vi "Terminal-Modbus-GetRead.vi"(0 "GuiModbusQRef":refnum<queue>, 11 "error in (no error)":errorcluster caption="错误输入（无错误）") -> (3 "液压子系统":u16[](array[numeric]), 4 "齿轮子系统-PLC":u16[](array[numeric]), 6 "齿轮子系统-数显表":u16[](array[numeric]), 8 "动力子系统-PLC":u16[](array[numeric]), 10 "动力子系统-温度巡检仪":u16[](array[numeric]), 14 "NI工控机":u16[](array[numeric]), 15 "error out":errorcluster caption="错误输出")   [LabVIEW 2014]
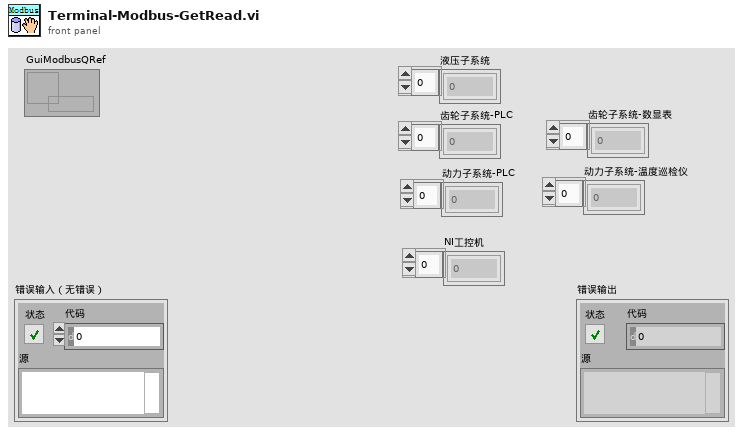
[diagram p1: front panel]
types:
  T1 = cluster{"Transaction ID":u16, "Unit ID":u8, "Starting Address":u16, "Quantity":u16, "Holding Registers":u16[], "Exception Code":u8}
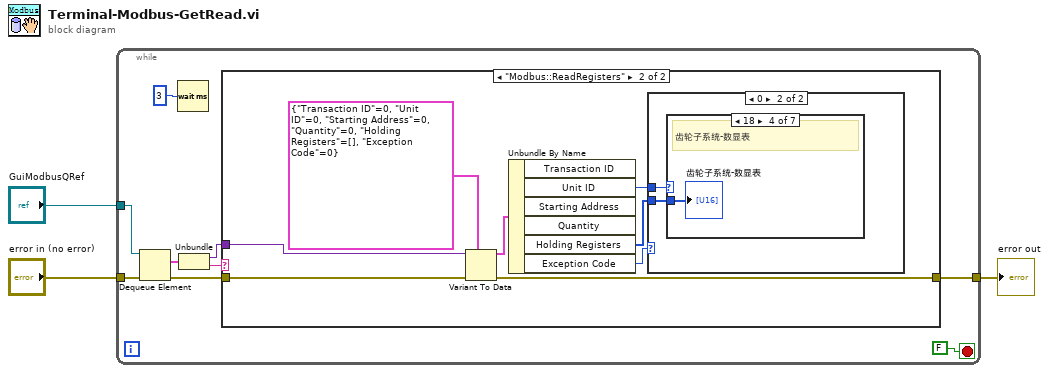
[diagram p0: block diagram]
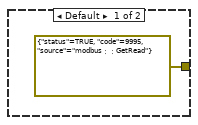
[diagram p2: hidden frame]
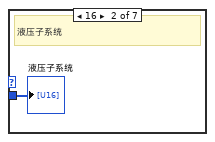
[diagram p5: hidden frame]
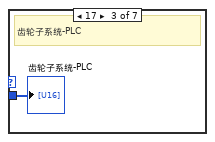
[diagram p6: hidden frame]
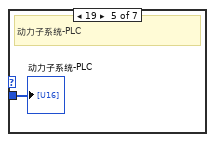
[diagram p7: hidden frame]
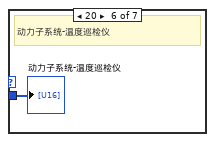
[diagram p8: hidden frame]
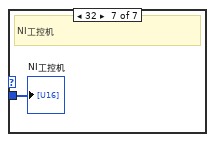
[diagram p9: hidden frame]
diagram:
  n1 = while {
    tunnel: "GuiModbusQRef" -> [w12]
    tunnel: "error in (no error)" -> [w11]
    tunnel: [w6] -> w1
    stop <- FALSE stop-if-true
    n2 = Dequeue Element(queue=w12, error in (no error)=w11) -> (element=w10:cluster{"Data":variant, "State":string}, error out=w7:errorcluster)  [unwired: 1 in, 2 out]
    n3 = Wait (ms)(milliseconds to wait=u32 3 ("等待时间（毫秒）")) -> ()  [unwired: 1 out]
    n4 = Unbundle(w10) -> ("Data"=w8:variant, "State"=w9:string)
    n5 = case shown="\"Modbus::ReadRegisters\"" w9 {
      tunnel: w8 -> [_ w21]
      tunnel: w7 -> [_ w20]
      tunnel: [errorcluster {"status"=TRUE, "code"=9995, "source"="modbus：：GetRead"} ("错误常量") w15] -> w6
      frame Default {
      }
      frame "Modbus::ReadRegisters" {
        n6 = Variant To Data(error in=w20, type=T1 {"Transaction ID"=0, "Unit ID"=0, "Starting Address"=0, "Quantity"=0, "Holding Registers"=[], "Exception Code"=0} ("元素"), Variant=w21) -> (data=w19:T1, error out=w15:errorcluster)
        n7 = Unbundle By Name(w19) -> ("Unit ID"=w16:u8, "Holding Registers"=w14:u16[], "Exception Code"=w17:u8)  [unwired: 3 out]
        n8 = case shown="0" w17 {
          tunnel: w16 -> [_ w23]
          tunnel: w14 -> [_ w22]
          frame Default {
          }
          frame 0 {
            n9 = case shown="18" w23 {
              tunnel: w22 -> [_ w24 w25 w26 w27 w28 w29]
              frame Default {
              }
              frame 16 {
                # "液压子系统"
                "液压子系统" <- w24
              }
              frame 17 {
                # "齿轮子系统-PLC"
                "齿轮子系统-PLC" <- w25
              }
              frame 18 {
                # "齿轮子系统-数显表"
                "齿轮子系统-数显表" <- w26
              }
              frame 19 {
                # "动力子系统-PLC"
                "动力子系统-PLC" <- w27
              }
              frame 20 {
                # "动力子系统-温度巡检仪"
                "动力子系统-温度巡检仪" <- w28
              }
              frame 32 {
                # "NI工控机"
                "NI工控机" <- w29
              }
            }
          }
        }
      }
    }
  }
  "error out" <- w1
